vi "UserName.vi"() -> ()   [LabVIEW 2017]
panel:
  in  "Home Button":bool=TRUE
  out "Waveform Chart":cluster{dbl, dbl, dbl}(graph)
  out "Table":string[][](table)
  in  "Stop":bool
  out "Result":string
  in  "Play Button":bool=TRUE
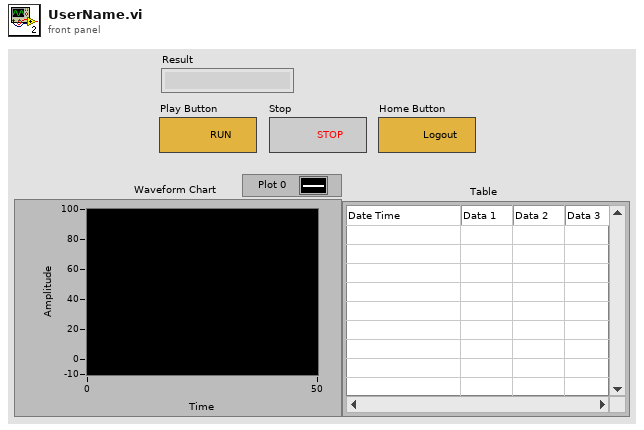
[diagram p1: front panel]
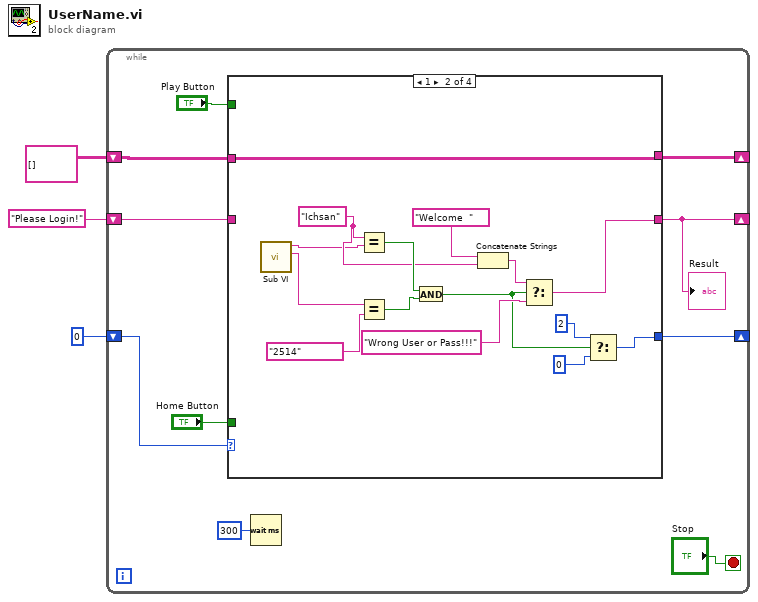
[diagram p0: block diagram]
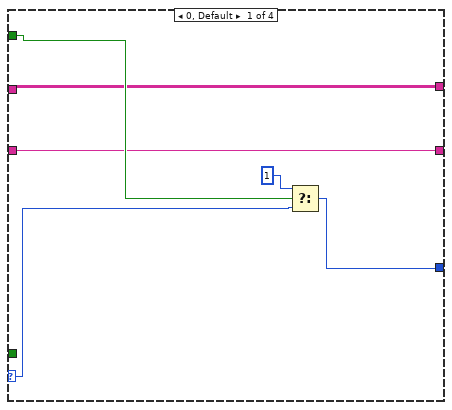
[diagram p2: hidden frame]
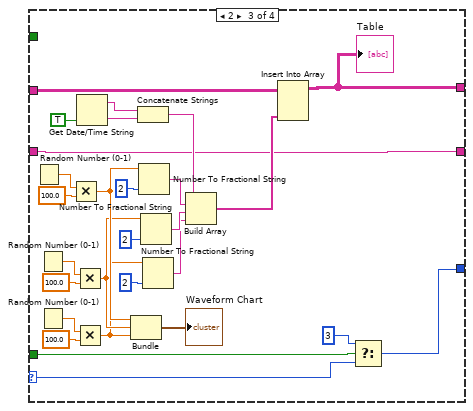
[diagram p3: hidden frame]
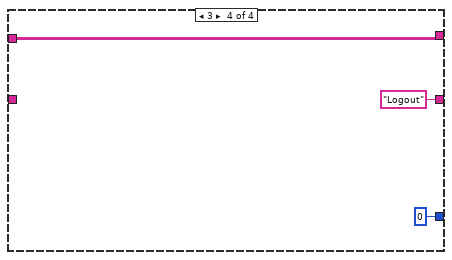
[diagram p4: hidden frame]
diagram:
  n1 = while {
    shift-right: [w13] -> _
    shift-left: 0 -> [w7]
    shift-right: [w9] -> _
    shift-left: string[][] [] -> [w10]
    shift-right: [w6] -> _
    shift-left: "Please Login!" ("String") -> [w5]
    stop <- "Stop" stop-if-true
    n2 = case shown="1" w7 {
      selector: w7 -> [w17 _ w37 _]
      tunnel: [w19 w34 w39 0] -> w13
      tunnel: "Play Button" -> [w18 _ _ _]
      tunnel: w10 -> [w15 w21 w46 w65]
      tunnel: [w15 w21 w40 w65] -> w9
      tunnel: "Home Button" -> [_ _ w36 _]
      tunnel: [w14 w20 w35 "Logout" ("String")] -> w6
      tunnel: w5 -> [w14 _ w35 _]
      frame 0, Default {
        n3 = Select(t=1, s=w18, f=w17) -> (s? t:f=w19:i32)
      }
      frame 1 {
        w24 = "Ichsan"
        n4 = call "Sub VI.vi"() -> ("Password 2"=w22:string, "User Name 2"=w23:string)  [unwired: 9 in, 1 out]
        n5 = Equal?(x=w24, y=w23) -> (x = y?=w27:bool)
        n6 = Equal?(x=w22, y="2514") -> (x = y?=w26:bool)
        n7 = And(x=w27, y=w26) -> (x .and. y?=w28:bool)
        n8 = Concatenate Strings("Welcome  ", w24) -> (w31:string)
        n9 = Select(t=w31, s=w28, f="Wrong User or Pass!!!") -> (s? t:f=w20:string)
        n10 = Select(t=2, s=w28, f=0) -> (s? t:f=w34:i32)
      }
      frame 2 {
        n11 = Random Number (0-1)() -> (number: 0 to 1=w60:dbl)
        n12 = Random Number (0-1)() -> (number: 0 to 1=w62:dbl)
        n13 = Random Number (0-1)() -> (number: 0 to 1=w58:dbl)
        n14 = Multiply(x=w60, y=100.0) -> (x*y=w44:dbl)
        n15 = Multiply(x=w62, y=100.0) -> (x*y=w43:dbl)
        n16 = Multiply(x=w58, y=100.0) -> (x*y=w42:dbl)
        n17 = Get Date/Time String(want seconds? (F)=TRUE) -> (date string=w56:string, time string=w55:string)  [unwired: 2 in]
        n18 = Bundle(w44, w43, w42) -> (→"Waveform Chart":cluster{dbl, dbl, dbl})  [unwired: 1 in]
        n19 = Concatenate Strings(w56, w55) -> (w54:string)
        n20 = Number To Fractional String(number=w44, precision (6)=2) -> (F-format string=w49:string)  [unwired: 2 in]
        n21 = Number To Fractional String(number=w43, precision (6)=2) -> (F-format string=w48:string)  [unwired: 2 in]
        n22 = Number To Fractional String(number=w42, precision (6)=2) -> (F-format string=w47:string)  [unwired: 2 in]
        n23 = Build Array(w54, w49, w48, w47) -> (w45:string[])
        n24 = Insert Into Array(array=w46, new element=w45) -> (w40:string[][])  [unwired: 2 in]
        "Table" <- w40
        n25 = Select(t=3, s=w36, f=w37) -> (s? t:f=w39:i32)
      }
      frame 3 {
      }
    }
    "Result" <- w6
    n26 = Wait (ms)(milliseconds to wait=u32 300) -> ()  [unwired: 1 out]
  }
